vi "Get Blob Snapshot Properties.vi"(7 "Snapshot":string, 8 "error in (no error)":errorcluster, 9 "Blob":string, 10 "Container":string, 11 "Azure Session in":refnum<class "Session.lvclass">) -> (0 "error out":errorcluster, 2 "Blob Properties":T1[](array[typedef]), 3 "Azure Session out":refnum<class "Session.lvclass">)   [LabVIEW 2015, in "NI_Azure_Blob.lvlib"]
doc: "Returns all system properties and user-defined metadata on a snapshot of a blob."
uses:
  NI_Azure_Blob.lvlib
  Core/Session/Session.lvclass
  Core/Name Value Pair.ctl
  Core/Session/Session.lvclass/Session.ctl
  Core/Session/Write HTTP Verb.vi
  Core/Session/Write URL Suffix.vi
  Core/Session/Write Request Parameters.vi
  Core/NI_Azure_Core.lvlib
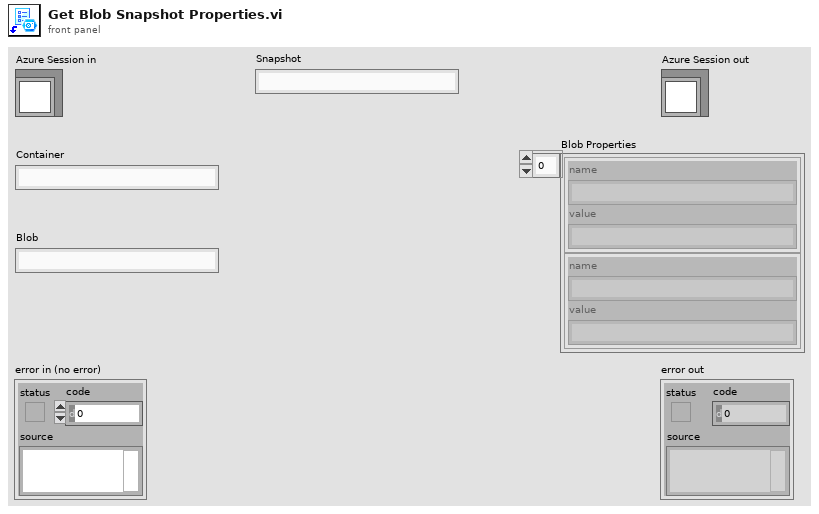
[diagram p1: front panel]
types:
  T1 = typedef "NI_Azure_Core.lvlib/Name Value Pair.ctl" = cluster{"name":string, "value":string}
  T2 = typedef "NI_Azure_Core.lvlib/Response.ctl" = cluster{"Headers":string, "Body":string}
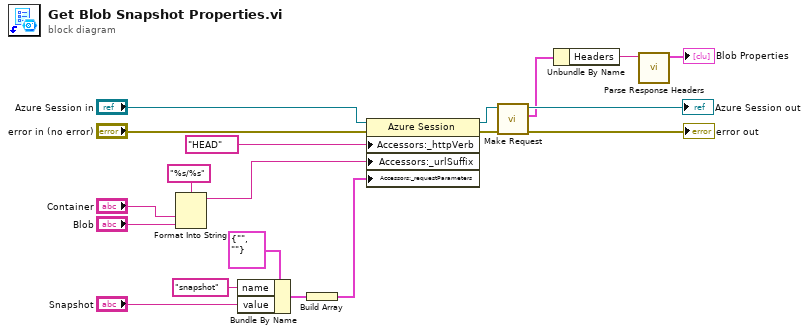
[diagram p0: block diagram]
diagram:
  n1 = Format Into String(format string="%s/%s", "Container", "Blob") -> (resulting string=w7:string)  [unwired: 2 in, 1 out]
  n2 = Bundle By Name(cluster=T1 {"name"="", "value"=""} ("Name Value Pair"), "name"="snapshot", "value"="Snapshot") -> (w3:T1)
  n3 = Build Array(w3) -> (w1:T1[])
  n4 = property class="Azure Session"(reference="Azure Session in", error in="error in (no error)", "Accessors:_httpVerb"="HEAD" ("HTTP-Verb"), "Accessors:_urlSuffix"=w7, "Accessors:_requestParameters"=w1) -> (reference out=w8:refnum<class "Session.lvclass">, error out=w10:errorcluster)
  n5 = call "Make Request.vi"("error in (no error)"=w10, "Session in"=w8) -> ("error out"=→"error out":errorcluster, "Response"=w11:T2, "Session out"=→"Azure Session out":refnum<class "Session.lvclass">)  [unwired: 7 in]
  n6 = Unbundle By Name(w11) -> ("Headers"=w13:string)
  n7 = call "Parse Response Headers.vi"("String"=w13) -> ("Response Headers"=→"Blob Properties":T1[])  [unwired: 10 in]
